vi "Down Sample Array.vi"(8 "Error in (no error)":errorcluster, 10 "Desired Sampling Rate":dbl=2000.0, 11 "Waveform Array":dbl[](array[numeric])) -> (0 "Error Out":errorcluster, 3 "Output Array":dbl[](array[numeric]))   [LabVIEW 2020]
doc: "This VI takes oversampled data and averages the data to downsample to the desired sampling rate. For instance, if data is captured at 2000 Hz for 1 second and the desired sampling rate is 50 Hz, every new data point is the result of averaging 40 data points (from the 2000 Hz data stream)."
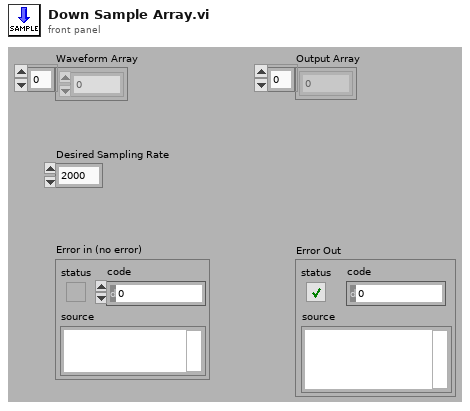
[diagram p1: front panel]
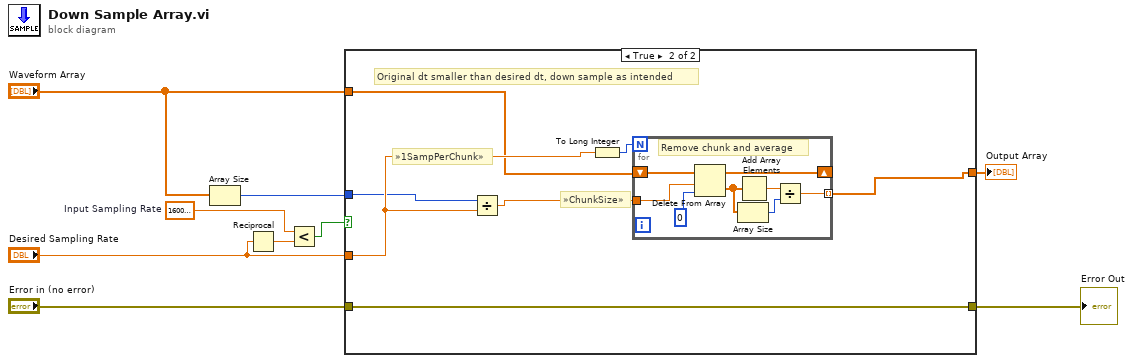
[diagram p0: block diagram]
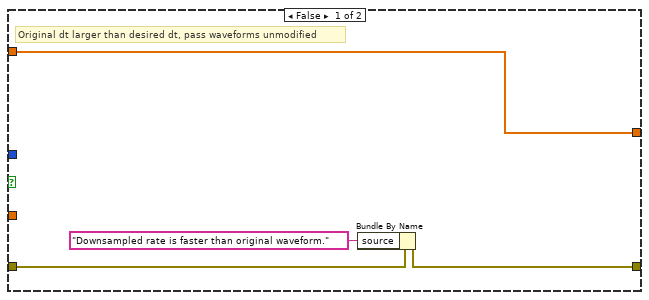
[diagram p2: hidden frame]
diagram:
  w2 = 1600000000.0  # Input Sampling Rate
  n1 = Array Size(array="Waveform Array") -> (size(s)=w9:i32)
  n2 = Reciprocal(x="Desired Sampling Rate") -> (1/x=w6:dbl)
  n3 = Less?(x=w2, y=w6) -> (x < y?=w5:bool)
  n4 = case shown="True" w5 {
    tunnel: "Desired Sampling Rate" -> [_ w19]
    tunnel: [w13 w15] -> w1
    tunnel: "Waveform Array" -> [w13 w18]
    tunnel: w9 -> [_ w17]
    tunnel: [w11 w16] -> w4
    tunnel: "Error in (no error)" -> [w12 w16]
    frame False {
      # "Original dt larger than desired dt, pass waveforms unmodified"
      n5 = Bundle By Name(cluster=w12, "source"="Downsampled rate is faster than original waveform.") -> (w11:errorcluster)
    }
    frame True {
      # "»ChunkSize»"
      # "Original dt smaller than desired dt, down sample as intended"
      # "»1SampPerChunk»"
      n6 = Divide(x=w17, y=w19) -> (x/y=w20:dbl)
      n7 = To Long Integer(number=w19) -> (32bit integer=w14:i32)
      n8 = for {
        N: w14 -> [_]
        tunnel: [w28] -> w15 mode=indexing
        shift-right: [w24] -> _
        shift-left: w18 -> [w25]
        tunnel: w20 -> [w23]
        # "Remove chunk and average"
        n9 = Delete From Array(array=w25, length=w23, index=0) -> (deleted portion=w22:dbl[], array with subset deleted=w24:dbl[])
        n10 = Array Size(array=w22) -> (size(s)=w21:i32)
        n11 = Add Array Elements(numeric array=w22) -> (sum=w27:dbl)
        n12 = Divide(x=w27, y=w21) -> (x/y=w28:dbl)
      }
    }
  }
  "Error Out" <- w4
  "Output Array" <- w1
